vi "host.vi"() -> ()   [LabVIEW 2020]
uses:
  <vilib>/FPGAPlugInAG/cRIO-9035/niLvFpga_Open_cRIO-9035.vi
  <vilib>/Utility/error.llb/Error Cluster From Error Code.vi
  <vilib>/rvi/errors/niLvFpgaAdjustHostInterfaceError.vi
  <vilib>/FPGAPlugInAG/cRIO-9035/niLvFpga_Run_cRIO-9035.vi
  <vilib>/FPGAPlugInAG/cRIO-9035/niLvFpga_Close_cRIO-9035.vi
  <vilib>/rvi/interface/nirviOpenFPGA/nirviOpenFPGA.xnode
  FPGA Bitfiles/labviewfpgacheck_FPGATarget_target_0Dyt68Qj0bU.lvbitx
  target.vi
  <vilib>/rvi/interface/nirviMethod/nirviMethod.xnode
  <vilib>/rvi/interface/nirviReadWriteControl/nirviReadWriteControl.xnode
  <vilib>/rvi/interface/nirviCloseFPGA/nirviCloseFPGA.xnode
  <vilib>/rvi/errors/niLvFpgaMergeErrorWithErrorCode.vi
  <vilib>/FPGAPlugInAG/cRIO-9035/niLvFpga_WriteFifo_cRIO-9035.vi
  NiFpgaLv.dll
  <vilib>/FPGAPlugInAG/cRIO-9035/niLvFpga_ReadFifo_cRIO-9035.vi
panel:
  out "A Sorted":sgl[](graph)
  out "A":sgl[](graph)
  out "time (ms)":dbl
  out "tick count":u32
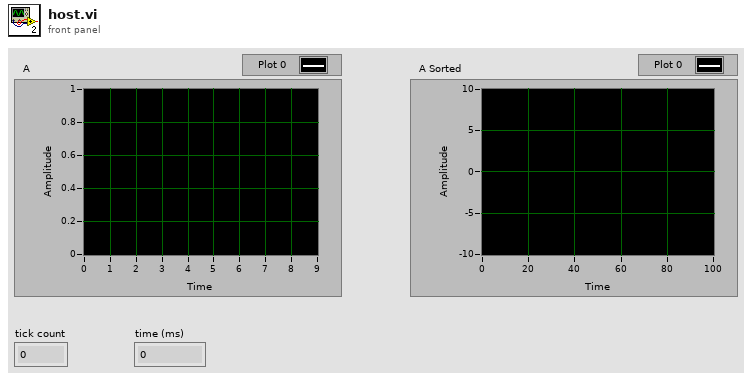
[diagram p1: front panel]
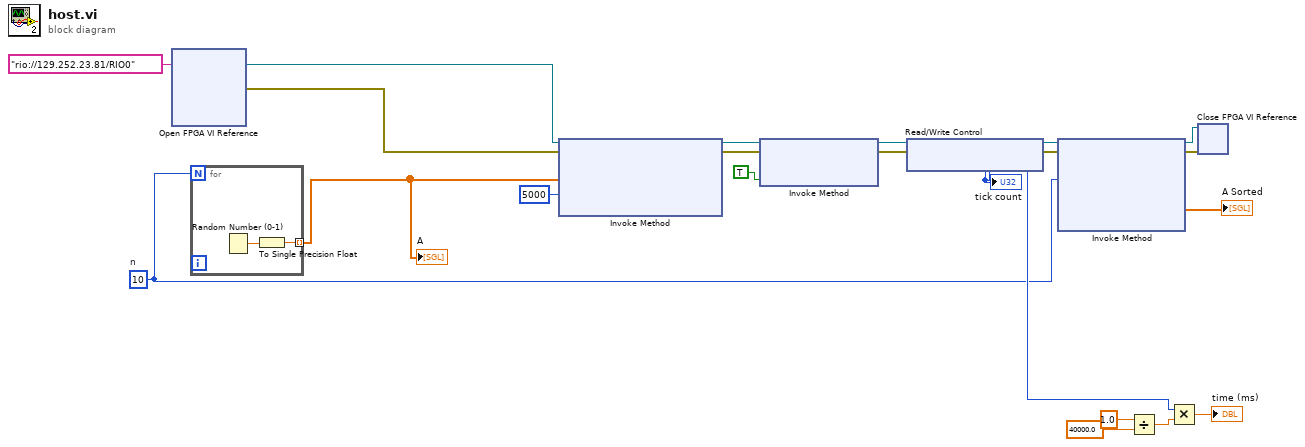
[diagram p0: block diagram]
diagram:
  w5 = 10  # n
  n1 = xnode "Open FPGA VI Reference"("resource name"=tag "rio://129.252.23.81/RIO0") -> ("FPGA VI Reference Out"=w3:refnum<k20>, "error out"=w2:errorcluster)  [unwired: 1 in]
  n2 = for {
    N: w5 -> [_]
    tunnel: [w22] -> w6 mode=indexing
    n3 = Random Number (0-1)() -> (number: 0 to 1=w23:dbl)
    n4 = To Single Precision Float(number=w23) -> (single precision float=w22:sgl)
  }
  "A" <- w6
  n5 = xnode "Invoke Method"("FPGA VI Reference In"=w3, "error in"=w2, "Data"=w6, "Timeout (ms)"=5000) -> ("FPGA VI Reference Out"=w18:refnum<k20>, "error out"=w17:errorcluster)  [unwired: 1 out]
  n6 = xnode "Invoke Method"("FPGA VI Reference In"=w18, "error in"=w17, "Wait Until Done (F)"=TRUE) -> ("FPGA VI Reference Out"=w16:refnum<k20>, "error out"=w15:errorcluster)
  n7 = xnode "Read/Write Control"("FPGA VI Reference In"=w16, "error in"=w15) -> ("FPGA VI Reference Out"=w14:refnum<k20>, "error out"=w13:errorcluster, "tick count"=w9:u32)
  "tick count" <- w9
  n8 = xnode "Invoke Method"("FPGA VI Reference In"=w14, "error in"=w13, "Number of Elements"=w5) -> ("FPGA VI Reference Out"=w20:refnum<k20>, "error out"=w19:errorcluster, "Data"=→"A Sorted":sgl[])  [unwired: 1 in, 1 out]
  n9 = Divide(x=1.0, y=40000.0) -> (x/y=w10:dbl)
  n10 = Multiply(x=w9, y=w10) -> (x*y=→"time (ms)":dbl)
  n11 = xnode "Close FPGA VI Reference"("FPGA VI Reference In"=w20, "error in"=w19) -> ()  [unwired: 1 out]
